vi "UIGetFlaggedRefsOnPane.vi"(6 "Check Flag (T)":bool=TRUE, 8 "error in":errorcluster, 9 "Flag":string="DATA-", 10 "VI Ref":refnum<vi>, 11 "UI Ref cluster in":T1) -> (0 "error out":errorcluster, 3 "UI Ref cluster out":T1)   [LabVIEW 2025, in "UI_Library.lvlib" / "UI_Library.lvclass"]
doc: "Get all VI Controls info: Label, Reference and DataType\nThe Controls can be filtered by using the FLAG label"
uses:
  UI_Library.lvclass
  Controls/UI_RefCluster.ctl
  <vilib>/Utility/Data Type/Type Definitions/Data Type.ctl
  <vilib>/Utility/Data Type/NI_Data Type.lvlib
  UI_Library.lvlib
panel:
  in  "DATA-String":string
  in  "DATA-Boolean":bool
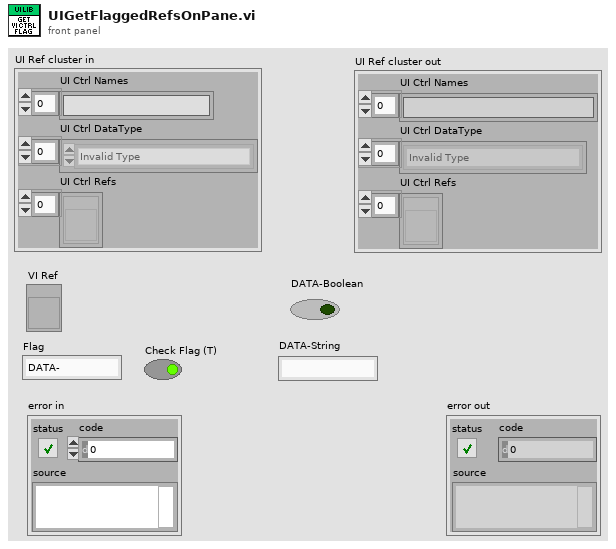
[diagram p1: front panel]
types:
  T1 = typedef "UI_Library.lvlib/UI_RefCluster.ctl" = cluster{"UI Ctrl Names":string[], "UI Ctrl DataType":T2[], "UI Ctrl Refs":refnum<vi>[]}
  T2 = typedef "NI_Data Type.lvlib/Data Type.ctl" = enum8{"Invalid Type", "Void", "I8", "I16", "I32", "I64", "U8", "U16", "U32", "U64", "Single Float", "Double Float", "Extended Float", "Single Complex", "Double Complex", "Extended Complex", "Enum U8", "Enum U16", "Enum U32", "Enum U64", "Single Float With Unit", "Double Float With Unit", "Extended Float With Unit", "Single Complex with Unit", "Double Complex with Unit", "Extended Complex with Unit", "Boolean", "String", "Path", "Picture", "Tag", "Array", "Cluster", "Variant", "LV Variant", "Waveform", "Timestamp", "Digital Waveform", "Digital Data", "ExpressData", "Refnum", "External Data", "VI", "Poly VI", "LabVIEW Class Instance", "Fixed Point", "Set Collection", "Map Collection"}
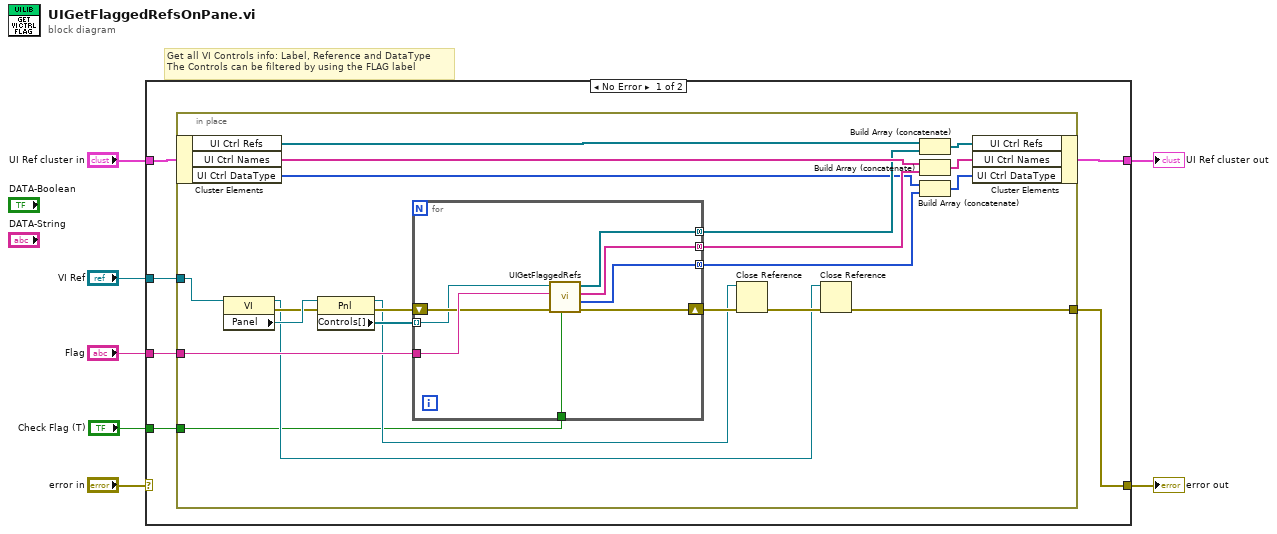
[diagram p0: block diagram]
diagram:
  # "Get all VI Controls info: Label, Reference and DataType\nThe Controls can be filtered by using the FLAG label"
  n1 = case shown="No Error" "error in" {
    selector: "error in" -> [_ w44]
    tunnel: "VI Ref" -> [w13 _]
    tunnel: [w12 w44] -> w5
    tunnel: "Flag" -> [w11 _]
    tunnel: "UI Ref cluster in" -> [w10 w43]
    tunnel: [w9 w43] -> w2
    tunnel: "Check Flag (T)" -> [w8 _]
    frame No Error {
      n2 = in-place "In Place Element Structure" {
        in-place-border: w13 -> [w14]
        in-place-border: [w18] -> w12
        in-place-border: w11 -> [w30]
        in-place-border: w8 -> [w15]
        n3 = in-place-cluster #1(w10) -> ("UI Ctrl Refs"=w27:refnum<vi>[], "UI Ctrl Names"=w26:string[], "UI Ctrl DataType"=w21:T2[])
        n4 = property on="Property Node" class="VI"(reference=w14) -> (reference out=w16:refnum<vi>, error out=w32:errorcluster, "Panel"=w34:refnum<vi>)  [unwired: 1 in]
        n5 = property on="Property Node" class="Pnl"(reference=w34, error in=w32) -> (reference out=w17:refnum<vi>, error out=w31:errorcluster, "Controls[]"=w33:refnum<vi>[])
        n6 = for {
          tunnel: w33 -> [w37] mode=indexing
          shift-right: [w36] -> w20
          shift-left: w31 -> [w39]
          tunnel: w30 -> [w42]
          tunnel: [w41] -> w25 mode=concatenating
          tunnel: [w40] -> w24 mode=concatenating
          tunnel: [w38] -> w22 mode=concatenating
          tunnel: w15 -> [w35]
          n7 = call "UIGetFlaggedRefs.vi"("Check Flag (T)"=w35, "error in"=w39, "Flag"=w42, "Control in"=w37) -> ("error out"=w36:errorcluster, "UI Ctrl DataType"=w38:T2[], "UI Ctrl Names"=w40:string[], "UI Ctrl Refs"=w41:refnum<vi>[])  [unwired: 4 in]
        }
        n8 = Close Reference(reference=w17, error in (no error)=w20) -> (error out=w19:errorcluster)
        n9 = Close Reference(reference=w16, error in (no error)=w19) -> (error out=w18:errorcluster)
        n10 = Build Array (concatenate)(w27, w25) -> (w29:refnum<vi>[])
        n11 = Build Array (concatenate)(w26, w24) -> (w28:string[])
        n12 = Build Array (concatenate)(w21, w22) -> (w23:T2[])
        n13 = in-place-cluster #1("UI Ctrl Refs"=w29, "UI Ctrl Names"=w28, "UI Ctrl DataType"=w23) -> (w9:T1)
      }
    }
    frame Error {
    }
  }
  "error out" <- w5
  "UI Ref cluster out" <- w2
